vi "Pockels Cal-Window size control.vi"(8 "error in (no error)":errorcluster, 9 "Function":T1, 11 "Original window size":cluster{"Horisontal":i16, "Vertical":i16}) -> (0 "error out":errorcluster)   [LabVIEW 2020]
uses:
  Typedefs/Colapsed-Expanded.ctl
  Globals/gl_Calibration globals.vi
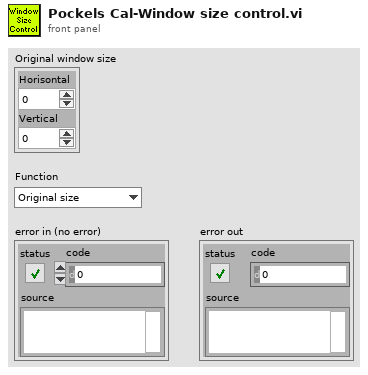
[diagram p1: front panel]
types:
  T1 = typedef "Colapsed-Expanded.ctl" = enum16{"Original size", "Expanded-Size A"}
  T2 = typedef "Pre-AOL Z wizard refs.ctl" = cluster{"VI's reference":refnum<vi>, "Calibration Mode":refnum<vi>, "Cal points":refnum<vi>, "Channel Selector":refnum<vi>, "Message":refnum<vi>, "Back":refnum<vi>, "Next":refnum<vi>, "Power meter AI":refnum<vi>, "2D Picture":refnum<vi>, "Note":refnum<vi>}
  T3 = typedef "LVRectTypeDef.ctl" = cluster{"Left":i16, "Top":i16, "Right":i16, "Bottom":i16}
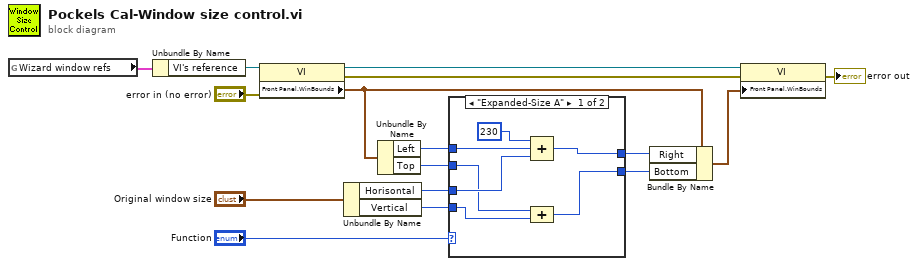
[diagram p0: block diagram]
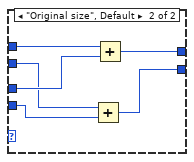
[diagram p2: hidden frame]
diagram:
  n1 = global read "gl_Calibration globals.vi" "Wizard window refs"() -> (w2:T2)
  n2 = Unbundle By Name(w2) -> ("VI's reference"=w1:refnum<vi>)
  n3 = property class="VI"(reference=w1, error in="error in (no error)") -> (reference out=w4:refnum<vi>, error out=w14:errorcluster, "Front Panel.WinBounds"=w6:T3)
  n4 = Unbundle By Name("Original window size") -> ("Horisontal"=w8:i16, "Vertical"=w11:i16)
  n5 = Unbundle By Name(w6) -> ("Left"=w7:i16, "Top"=w10:i16)
  n6 = case shown="\"Expanded-Size A\"" "Function" {
    tunnel: w7 -> [w23 w29]
    tunnel: w8 -> [w22 w28]
    tunnel: [w21 w27] -> w9
    tunnel: w10 -> [w20 w26]
    tunnel: w11 -> [w19 w25]
    tunnel: [w18 w24] -> w12
    frame "Expanded-Size A" {
      n7 = Compound Arithmetic op=ADD(i16 230 ("value"), w23, w22) -> (w21:i16)
      n8 = Compound Arithmetic op=ADD(w20, w19) -> (w18:i16)
    }
    frame "Original size", Default {
      n9 = Add(x=w26, y=w25) -> (x+y=w24:i16)
      n10 = Add(x=w29, y=w28) -> (x+y=w27:i16)
    }
  }
  n11 = Bundle By Name(cluster=w6, "Right"=w9, "Bottom"=w12) -> (w5:T3)
  n12 = property class="VI"(reference=w4, error in=w14, "Front Panel.WinBounds"=w5) -> (error out=→"error out":errorcluster)  [unwired: 1 out]
